vi "Check suspend.vi"(8 "Error In":errorcluster, 9 "Old data":T1={"Channels to measure"=[1.0], "Record heater"=FALSE, "Set point"=0.0, "Set Heater Range"=enum."Off", "Control"=FALSE, "Approach"=enum."Instant", "Ramp rate, K/min"=1.0, "Control Channel"=1, "P"=0.0, "I"=0.0, "D"=0.0, "Suspend heater"=FALSE}, 10 "New data":T1={"Channels to measure"=[1.0], "Record heater"=FALSE, "Set point"=0.0, "Set Heater Range"=enum."Off", "Control"=FALSE, "Approach"=enum."Instant", "Ramp rate, K/min"=1.0, "Control Channel"=1, "P"=0.0, "I"=0.0, "D"=0.0, "Suspend heater"=FALSE}, 11 "VISA resource name":refnum<visa-resource-name>) -> (0 "Error Out":errorcluster, 3 "VISA resource name out":refnum<visa-resource-name>)   [LabVIEW 2015]
uses:
  Neocera Front Panel Data.ctl
  Neocera Heater Ranges.ctl
  Neocera Set Point Aproach.ctl
panel:
  # "Temperature Monitor"
  # "Temperature Control"
  # "Temperature Monitor"
  # "Temperature Control"
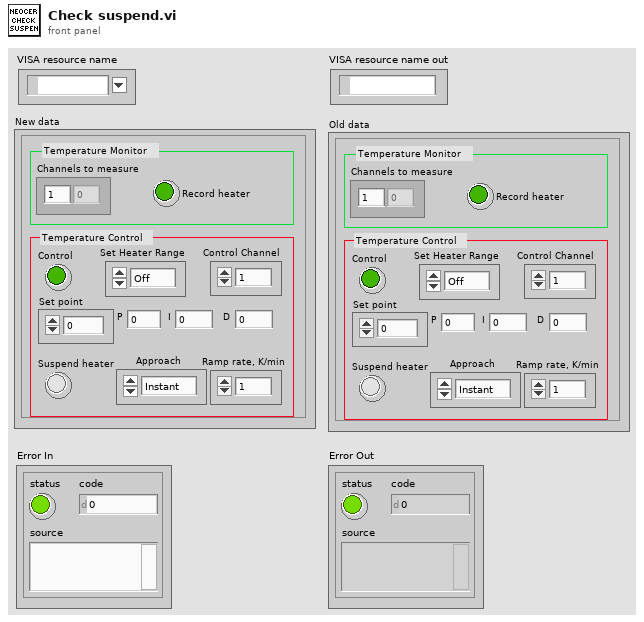
[diagram p1: front panel]
types:
  T1 = typedef "Neocera Front Panel Data.ctl" = cluster{"Channels to measure":dbl[], "Record heater":bool, "Set point":dbl, "Set Heater Range":T2, "Control":bool, "Approach":T3, "Ramp rate, K/min":dbl, "Control Channel":i16, "P":dbl, "I":dbl, "D":dbl, "Suspend heater":bool}
  T2 = typedef "Neocera Heater Ranges.ctl" = enum16{"Off", "0.05W", "0.5W", "5W", "50W"}
  T3 = typedef "Neocera Set Point Aproach.ctl" = enum16{"Instant", "Ramp"}
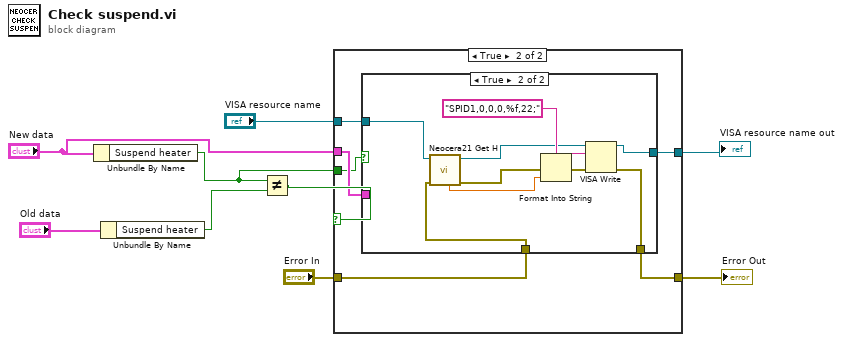
[diagram p0: block diagram]
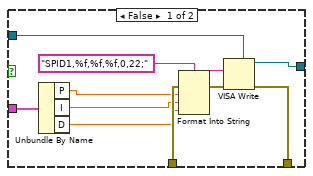
[diagram p3: hidden frame]
diagram:
  n1 = Unbundle By Name("New data") -> ("Suspend heater"=w1:bool)
  n2 = Unbundle By Name("Old data") -> ("Suspend heater"=w4:bool)
  n3 = Not Equal?(x=w1, y=w4) -> (x != y?=w3:bool)
  n4 = case shown="True" w3 {
    tunnel: "Error In" -> [w10 w17]
    tunnel: [w10 w14] -> w7
    tunnel: "VISA resource name" -> [w11 w16]
    tunnel: [w11 w15] -> w5
    tunnel: "New data" -> [_ w13]
    tunnel: w1 -> [_ w12]
    frame False {
    }
    frame True {
      n5 = case shown="True" w12 {
        tunnel: w17 -> [w27 w37]
        tunnel: w16 -> [w24 w38]
        tunnel: [w23 w29] -> w15
        tunnel: [w22 w31] -> w14
        tunnel: w13 -> [w21 _]
        frame False {
          n6 = Unbundle By Name(w21) -> ("P"=w20:dbl, "I"=w19:dbl, "D"=w18:dbl)
          n7 = Format Into String(format string="SPID1,%f,%f,%f,0,22;", error in=w27, w20, w19, w18) -> (resulting string=w25:string, error out=w26:errorcluster)  [unwired: 1 in]
          n8 = VISA Write(VISA resource name=w24, write buffer=w25, error in (no error)=w26) -> (VISA resource name out=w23:refnum<visa-resource-name>, error out=w22:errorcluster)  [unwired: 1 out]
        }
        frame True {
          n9 = call "Neocera21 Get H.vi"("error in (no error)"=w37, "VISA Resource Name"=w38) -> ("error out"=w33:errorcluster, "VISA Resource Name Out"=w30:refnum<visa-resource-name>, "Heat %"=w34:dbl)  [unwired: 4 in, 3 out]
          n10 = Format Into String(format string="SPID1,0,0,0,%f,22;", error in=w33, w34) -> (resulting string=w35:string, error out=w32:errorcluster)  [unwired: 1 in]
          n11 = VISA Write(VISA resource name=w30, write buffer=w35, error in (no error)=w32) -> (VISA resource name out=w29:refnum<visa-resource-name>, error out=w31:errorcluster)  [unwired: 1 out]
        }
      }
    }
  }
  "VISA resource name out" <- w5
  "Error Out" <- w7
